vi "Reset.vi"(11 "Test Handler in":refnum<class "Test Handler.lvclass">) -> (2 "successful?":bool, 3 "Test Handler out":refnum<class "Test Handler.lvclass">)   [LabVIEW 2018, in "Test Handler.lvclass"]
uses:
  Test Handler.lvclass
  Test Handler.lvclass/Test Handler.ctl
  <vilib>/Utility/config.llb/Read Key (Boolean).vi
  Utilities/Utilities.lvlib
  <vilib>/Utility/config.llb/NI_LVConfig.lvlib
panel:
  # "Connector Pane"
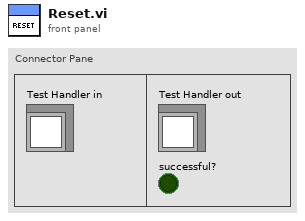
[diagram p1: front panel]
types:
  T1 = typedef "NI_LVConfig.lvlib/Config Data RefNum.ctl" = refnum<k1>
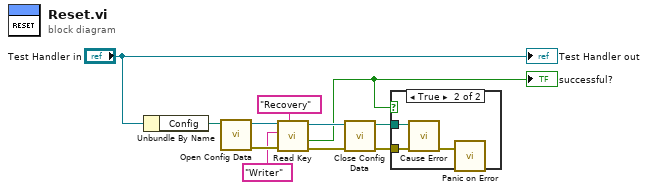
[diagram p0: block diagram]
diagram:
  n1 = Unbundle By Name("Test Handler in") -> ("Config"=w6:path)
  n2 = call <vilib>:"Open Config Data.vi"("configuration file path"=w6) -> ("error out"=w9:errorcluster, "refnum"=w10:T1)  [unwired: 8 in, 1 out]
  n3 = call-poly <vilib>:"Read Key.vi"("section"="Recovery" ("key"), "error in (no error)"=w9, "key"="Writer", "refnum"=w10) -> ("error out"=w2:errorcluster, "value"=w3:bool, "refnum out"=w5:T1)  [unwired: 4 in, 1 out]
  "successful?" <- w3
  n4 = call <vilib>:"Close Config Data.vi"("error in (no error)"=w2, "refnum"=w5) -> ("error out"=w1:errorcluster, "file path"=w4:path)  [unwired: 8 in]
  n5 = case shown="True" w3 {
    tunnel: w1 -> [_ w13]
    tunnel: w4 -> [_ w12]
    frame False {
    }
    frame True {
      n6 = call "Cause Error.vi"("error in (no error)"=w13, "ini file path"=w12) -> ("error out"=w14:errorcluster)  [unwired: 8 in, 1 out]
      n7 = call "Panic on Error.vi"("error in (no error)"=w14) -> ()  [unwired: 3 in]
    }
  }
  "Test Handler out" <- "Test Handler in"
